vi "Get_Wavelength.vi"(8 "error in (no error)":errorcluster, 11 "Abstract_Powermeter in":refnum<class "Abstract_Powermeter.lvclass">) -> (0 "error out":errorcluster, 2 "Wavelength (m)":dbl, 3 "Abstract_Powermeter out":refnum<class "Abstract_Powermeter.lvclass">)   [LabVIEW 2020, in "Abstract_Powermeter.lvclass"]
uses:
  <instrlib>/Classes/Powermeter/Abstract/Abstract_Powermeter.lvclass
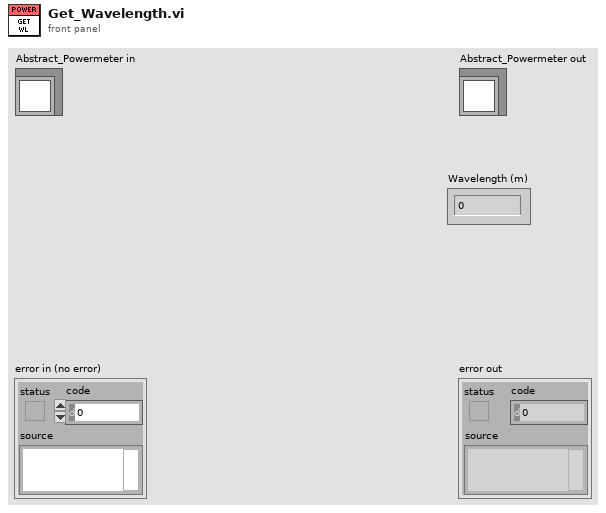
[diagram p1: front panel]
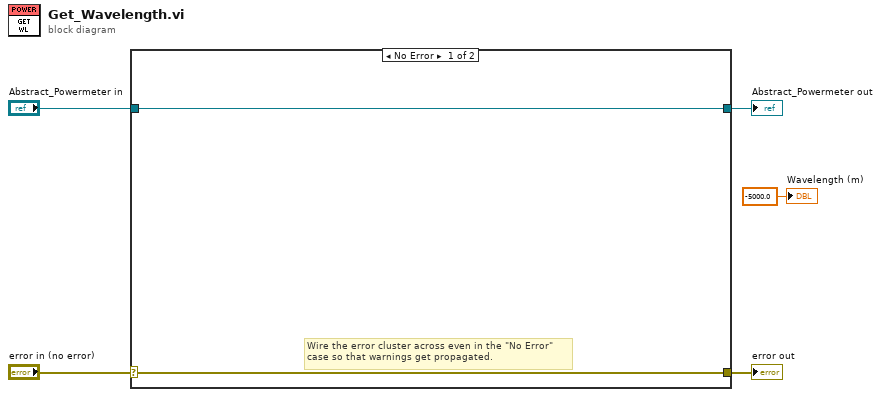
[diagram p0: block diagram]
diagram:
  n1 = case shown="No Error" "error in (no error)" {
    selector: "error in (no error)" -> [w6 w9]
    tunnel: [w6 w9] -> w4
    tunnel: [w7 w8] -> w2
    tunnel: "Abstract_Powermeter in" -> [w7 w8]
    frame No Error {
      # "Wire the error cluster across even in the \"No Error\"\ncase so that warnings get propagated."
    }
    frame Error {
    }
  }
  "error out" <- w4
  "Abstract_Powermeter out" <- w2
  "Wavelength (m)" <- -5000.0 ("Wavelength")
